vi "操作GRR表格.vi"(7 "表单":enum16{"0", "1", "2"}[](array[ring]), 8 "错误输入（无错误）":errorcluster, 9 "数据":string[](array[string]), 10 "位置":string[](array[string]), 11 "路径":path=path "C:/Users/Administrator/Desktop/GRR模板/Test.xlsx") -> (0 "错误输出":errorcluster, 2 "number":string, 3 "大小 2":i32)   [LabVIEW 2017]
panel:
  out "大小":i32
  out "数值":i32
  out "Worksheets":refnum<k7>
  out "Open":refnum<k7>
  in  "布尔":bool=TRUE
  in  "Excel._Application 2":refnum<k7>
  in  "Excel._Application":refnum<k7>
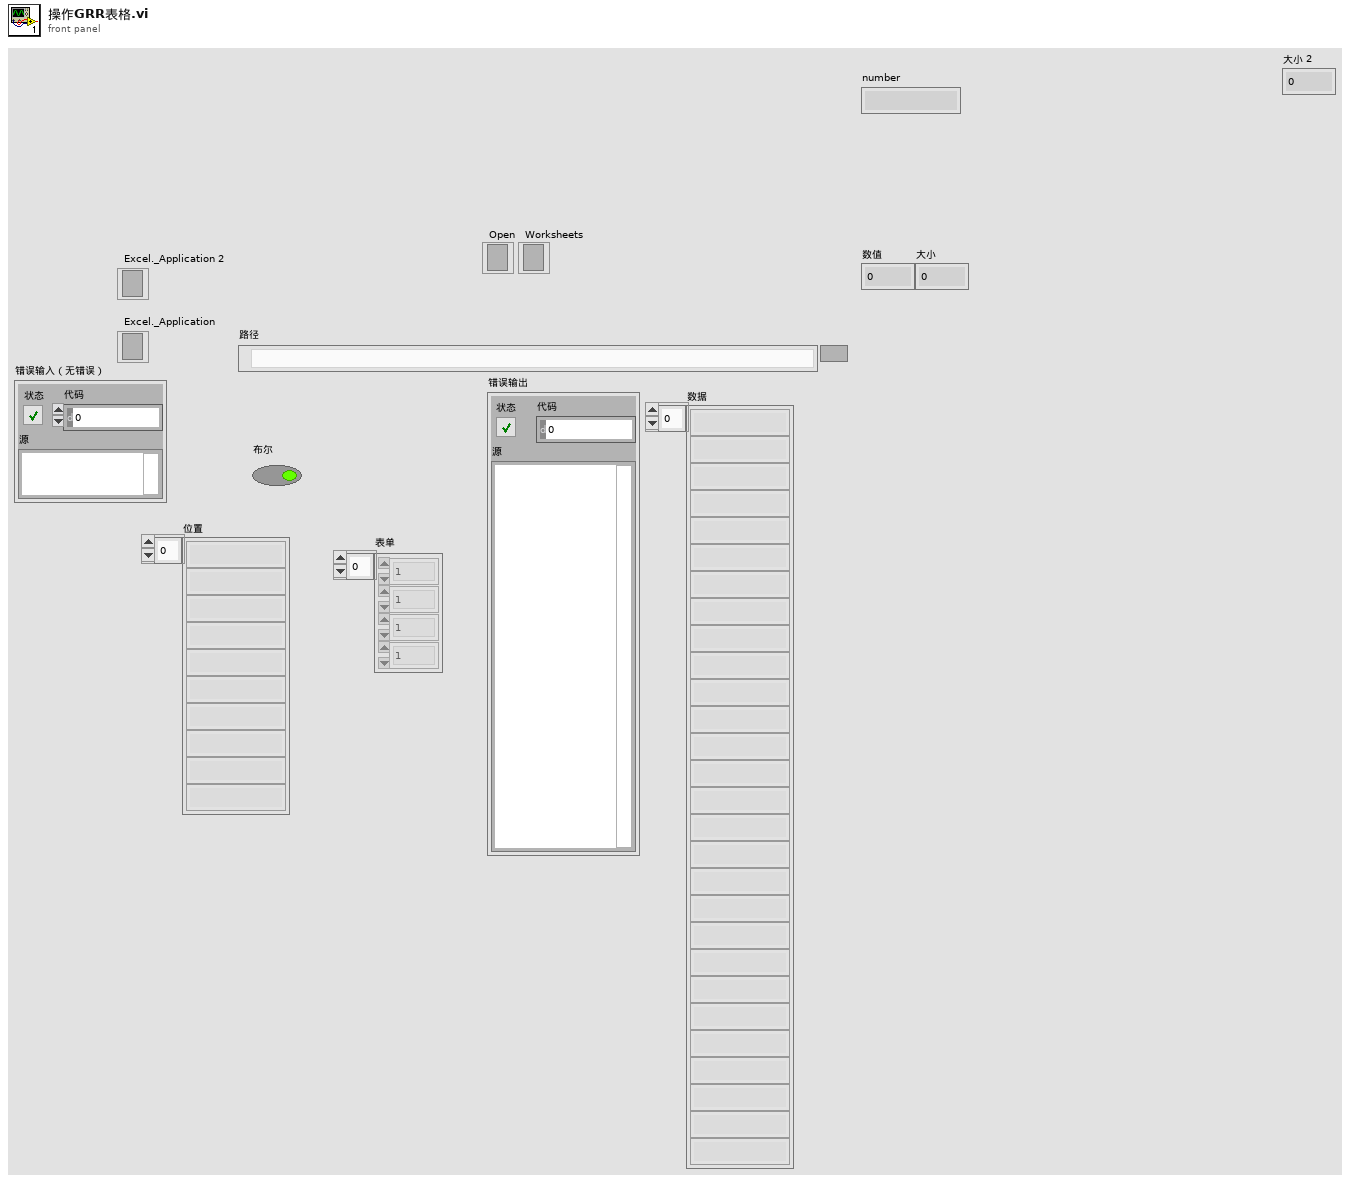
[diagram p1: front panel]
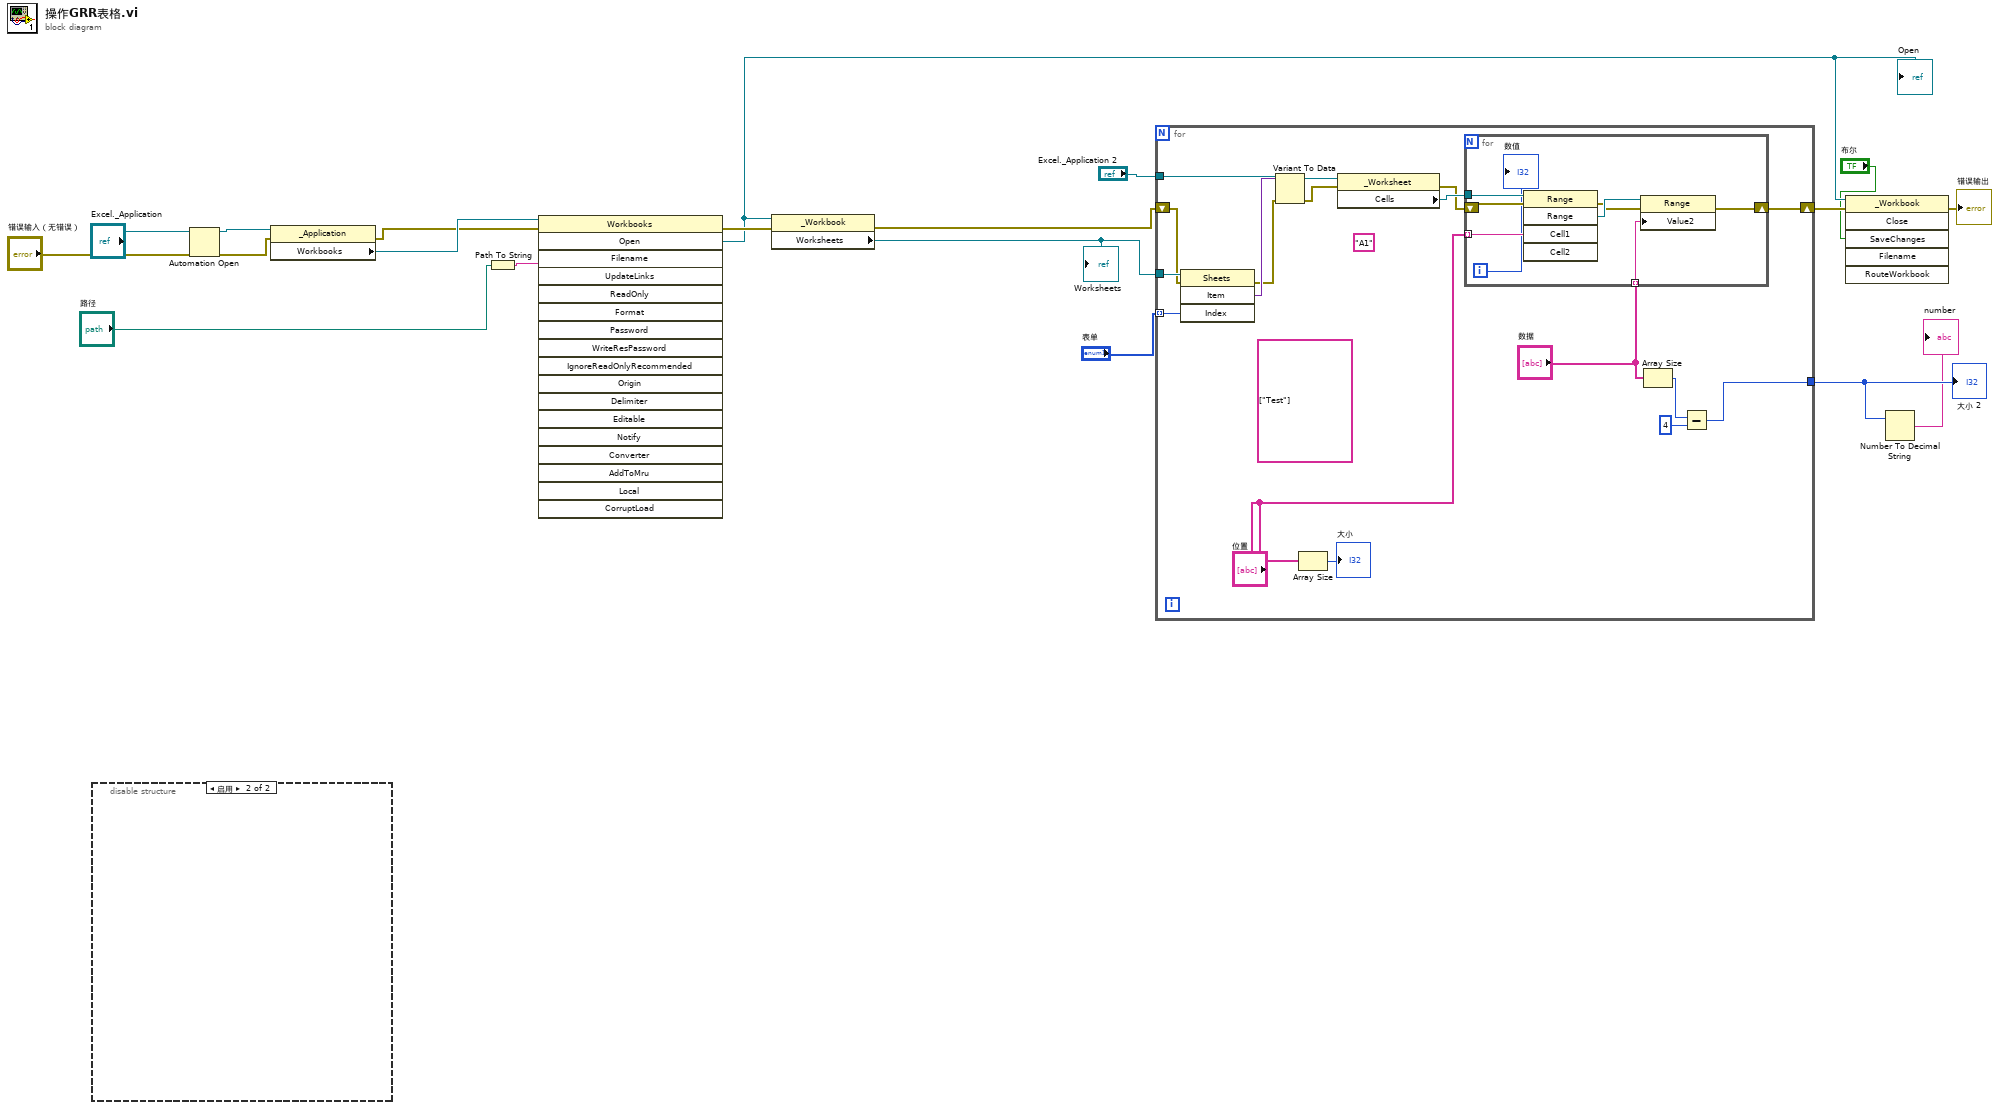
[diagram p0: block diagram]
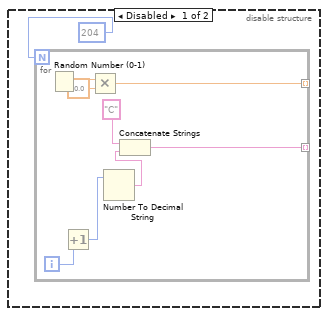
[diagram p2: hidden frame]
diagram:
  n1 = disable-structure shown="启用" {
    frame Disabled {
      n2 = for {
        N: 204 -> [_]
        tunnel: [w26] -> _ mode=indexing
        tunnel: [w21] -> _ mode=indexing
        i -> [w24]
        n3 = Random Number (0-1)() -> (number: 0 to 1=w28:dbl)
        n4 = Increment(x=w24) -> (x+1=w23:i32)
        n5 = Multiply(x=w28, y=10.0) -> (x*y=w26:dbl)
        n6 = Number To Decimal String(number=w23) -> (decimal integer string=w22:string)  [unwired: 1 in]
        n7 = Concatenate Strings("C", w22) -> (w21:string)
      }
    }
    frame Enabled {
    }
  }
  n8 = Automation Open(error in (no error)="错误输入（无错误）", Automation Refnum="Excel._Application") -> (Automation Refnum=w18:refnum<k7>, error out=w6:errorcluster)  [unwired: 2 in]
  n9 = property on="属性节点" class="_Application"(reference=w18, error in=w6) -> (error out=w14:errorcluster, "Workbooks"=w17:refnum<k7>)  [unwired: 1 out]
  n10 = Path To String(path="路径") -> (string=w15:string)
  n11 = invoke on="调用节点" class="Workbooks" method="Open"(reference=w17, error in=w14, "Filename"=w15) -> (error out=w11:errorcluster, "Open"=w9:refnum<k7>)  [unwired: 15 in, 16 out]
  "Open" <- w9
  n12 = property on="属性节点" class="_Workbook"(reference=w9, error in=w11) -> (error out=w10:errorcluster, "Worksheets"=w13:refnum<k7>)  [unwired: 1 out]
  "Worksheets" <- w13
  n13 = for {
    tunnel: w13 -> [w45]
    tunnel: "表单" -> [w44] mode=indexing
    tunnel: "Excel._Application 2" -> [w42]
    shift-right: [w35] -> w8
    shift-left: w10 -> [w39]
    tunnel: [w29] -> w2
    (unwired) string[] ["Test"]
    (unwired) "A1"
    n14 = invoke on="调用节点" class="Sheets" method="Item"(reference=w45, error in=w39, "Index"=w44) -> (error out=w38:errorcluster, "Item"=w43:variant)  [unwired: 1 in, 2 out]
    n15 = Variant To Data(error in=w38, type=w42, Variant=w43) -> (data=w41:refnum<k7>, error out=w37:errorcluster)
    n16 = Array Size(array="位置") -> (size(s)=→"大小":i32)
    n17 = property on="属性节点" class="_Worksheet"(reference=w41, error in=w37) -> (error out=w36:errorcluster, "Cells"=w40:refnum<k7>)  [unwired: 1 out]
    n18 = for {
      tunnel: w40 -> [w53]
      tunnel: "位置" -> [w52] mode=indexing
      tunnel: "数据" -> [w47] mode=indexing
      shift-right: [w48] -> w35
      shift-left: w36 -> [w50]
      i -> [w46]
      n19 = invoke on="调用节点" class="Range" method="Range"(reference=w53, error in=w50, "Cell1"=w52) -> (error out=w49:errorcluster, "Range"=w51:refnum<k7>)  [unwired: 2 in, 3 out]
      n20 = property on="属性节点" class="Range"(reference=w51, error in=w49, "Value2"=w47) -> (error out=w48:errorcluster)  [unwired: 1 out]
      "数值" <- w46
    }
    n21 = Array Size(array="数据") -> (size(s)=w30:i32)
    n22 = Subtract(x=w30, y=4) -> (x-y=w29:i32)
  }
  "大小 2" <- w2
  n23 = invoke on="调用节点" class="_Workbook" method="Close"(reference=w9, error in=w8, "SaveChanges"="布尔") -> (error out=→"错误输出":errorcluster)  [unwired: 3 in, 5 out]
  n24 = Number To Decimal String(number=w2) -> (decimal integer string=→"number":string)  [unwired: 1 in]
